vi "Main FPGA 5-axis with Limits and changes.vi"() -> ()   [LabVIEW 2013]
uses:
  <vilib>/Motion/MotorControl/_s/nism.interpretControlRegister.stateTransition.ctl
  <vilib>/Platform/TimedLoop/XDataNode/timing_clust.ctl
  <vilib>/Platform/TimedLoop/XDataNode/nitl_modes.ctl
  <vilib>/Platform/TimedLoop/XDataNode/wakeup.ctl
  <vilib>/Motion/MotorControl/_s/nism.digitalInputs.portA.ctl
  <vilib>/rvi/Emulation/niFpgaSctlEmulationGetInTimedLoop.vi
  <vilib>/rvi/Emulation/niFpgaEmulationReportErrorSimple.vi
  <vilib>/rvi/Emulation/niFpgaGetClockAttributes.vi
  <vilib>/rvi/Emulation/niFpgaCriticalErrorInLSC.vi
  Global FPGA.vi
  <vilib>/rvi/eio/common/nirviEmuTemplateMethod_errors.vi
  <vilib>/Motion/SoftMotion/Synchronization/nism.rioScan.generateSyncScan.vi
  <vilib>/rvi/Emulation/niFpgaProcessEmulError.vi
  <vilib>/Motion/MotorControl/_s/nism.interpretControlRegister.indexed.vi
  <vilib>/Motion/MotorControl/_s/nism.generateStatusRegister.indexed.vi
  <vilib>/Motion/MotorControl/_s/nism.mdo.read.dio.portA.2.vi
  <vilib>/Motion/MotorControl/_s/nism.mdo.read.positionLoopSyncData.vi
  <vilib>/Motion/MotorControl/_s/nism.mdo.read.splineData.vi
  <vilib>/Motion/MotorControl/_s/nism.splineInterpolation.fxp.3.index.vi
  <vilib>/Motion/MotorControl/_s/nism.mdo.handler.indexed.vi
  <vilib>/Motion/MotorControl/_s/nism.digitalFilter.u8.vi
  <vilib>/Motion/MotorControl/_s/nism.interpretDIOControl.portA.single.2.vi
  <vilib>/Motion/MotorControl/_s/nism.generateDIOStatus.portA.single.vi
  <vilib>/Platform/TimedLoop/XDataNode/XDataNode.xnode
  <vilib>/eio/EIONode/EIONode.xnode
  <vilib>/Motion/MotorControl/NI_SoftMotion_MotorControlIP.lvlib
  <vilib>/Platform/TimedLoop/XDataNode/XDNodeRunTimeDep.lvlib
  <vilib>/Motion/SoftMotion/Synchronization/NI_SoftMotion_Synchronization.lvlib
panel:
  in  "Axis Digital Inputs (U8)":u8[](array[numeric])=[0, 0, 0, 0, 0, 0, 0, 0]
  out "Axis Positions":fxp<+/-,64,32>[](array[numeric])
  in  "STEP or CW? (T=STEP)":bool
  out "Drive Enable":bool[](array[boolean])
  in  "Enable Watchdog":bool
  in  "Pet Watchdog":bool
  in  "Watchdog Timeout Period (ticks)":u64=40000000 format="%.0p"
  out "Watchdog Timed Out?":bool
  out "Time Since Last Pet":u64
  in  "Enable value":bool
  in  "Drive Enable override?":bool
  out "State":T1=enum."Start --> Initializing" caption="state transition"
  in  "Sync Value":bool
  in  "Sync Enable override?":bool
  in  "Invert direction?":bool
  out "Sync is Fault":bool
  out "Sync is Locked":bool
  in  "minimum pulse":u16=40
  # "Synchronization Loop"
  # "Control Status Loop"
  # "Notes: \n1. This VI provides the communication interface between the NI SoftMotion Engine and the LabVIEW FPGA Module. You must compile this VI for a specific FPGA target before use. After compiling, run the VI before running any of the Express VI examples. For information on moving this example to another FPGA target, refer to ni.com/info and enter info code fpgaex.\n\n2. Only use the Reset Axis button if you are unable to communicate with the axis by any other means. This button resets the device state machine and other VIs to a known state. After resetting the axis, switch the NI Scan Engine from Active Mode to Configuration Mode, then back to Active Mode, before attempting to enable the axis."
  # "(These two buttons \nare for testing\npurposes.)"
  # "(These two buttons \nare for testing\npurposes.)"
  # "Step/Direction Loop"
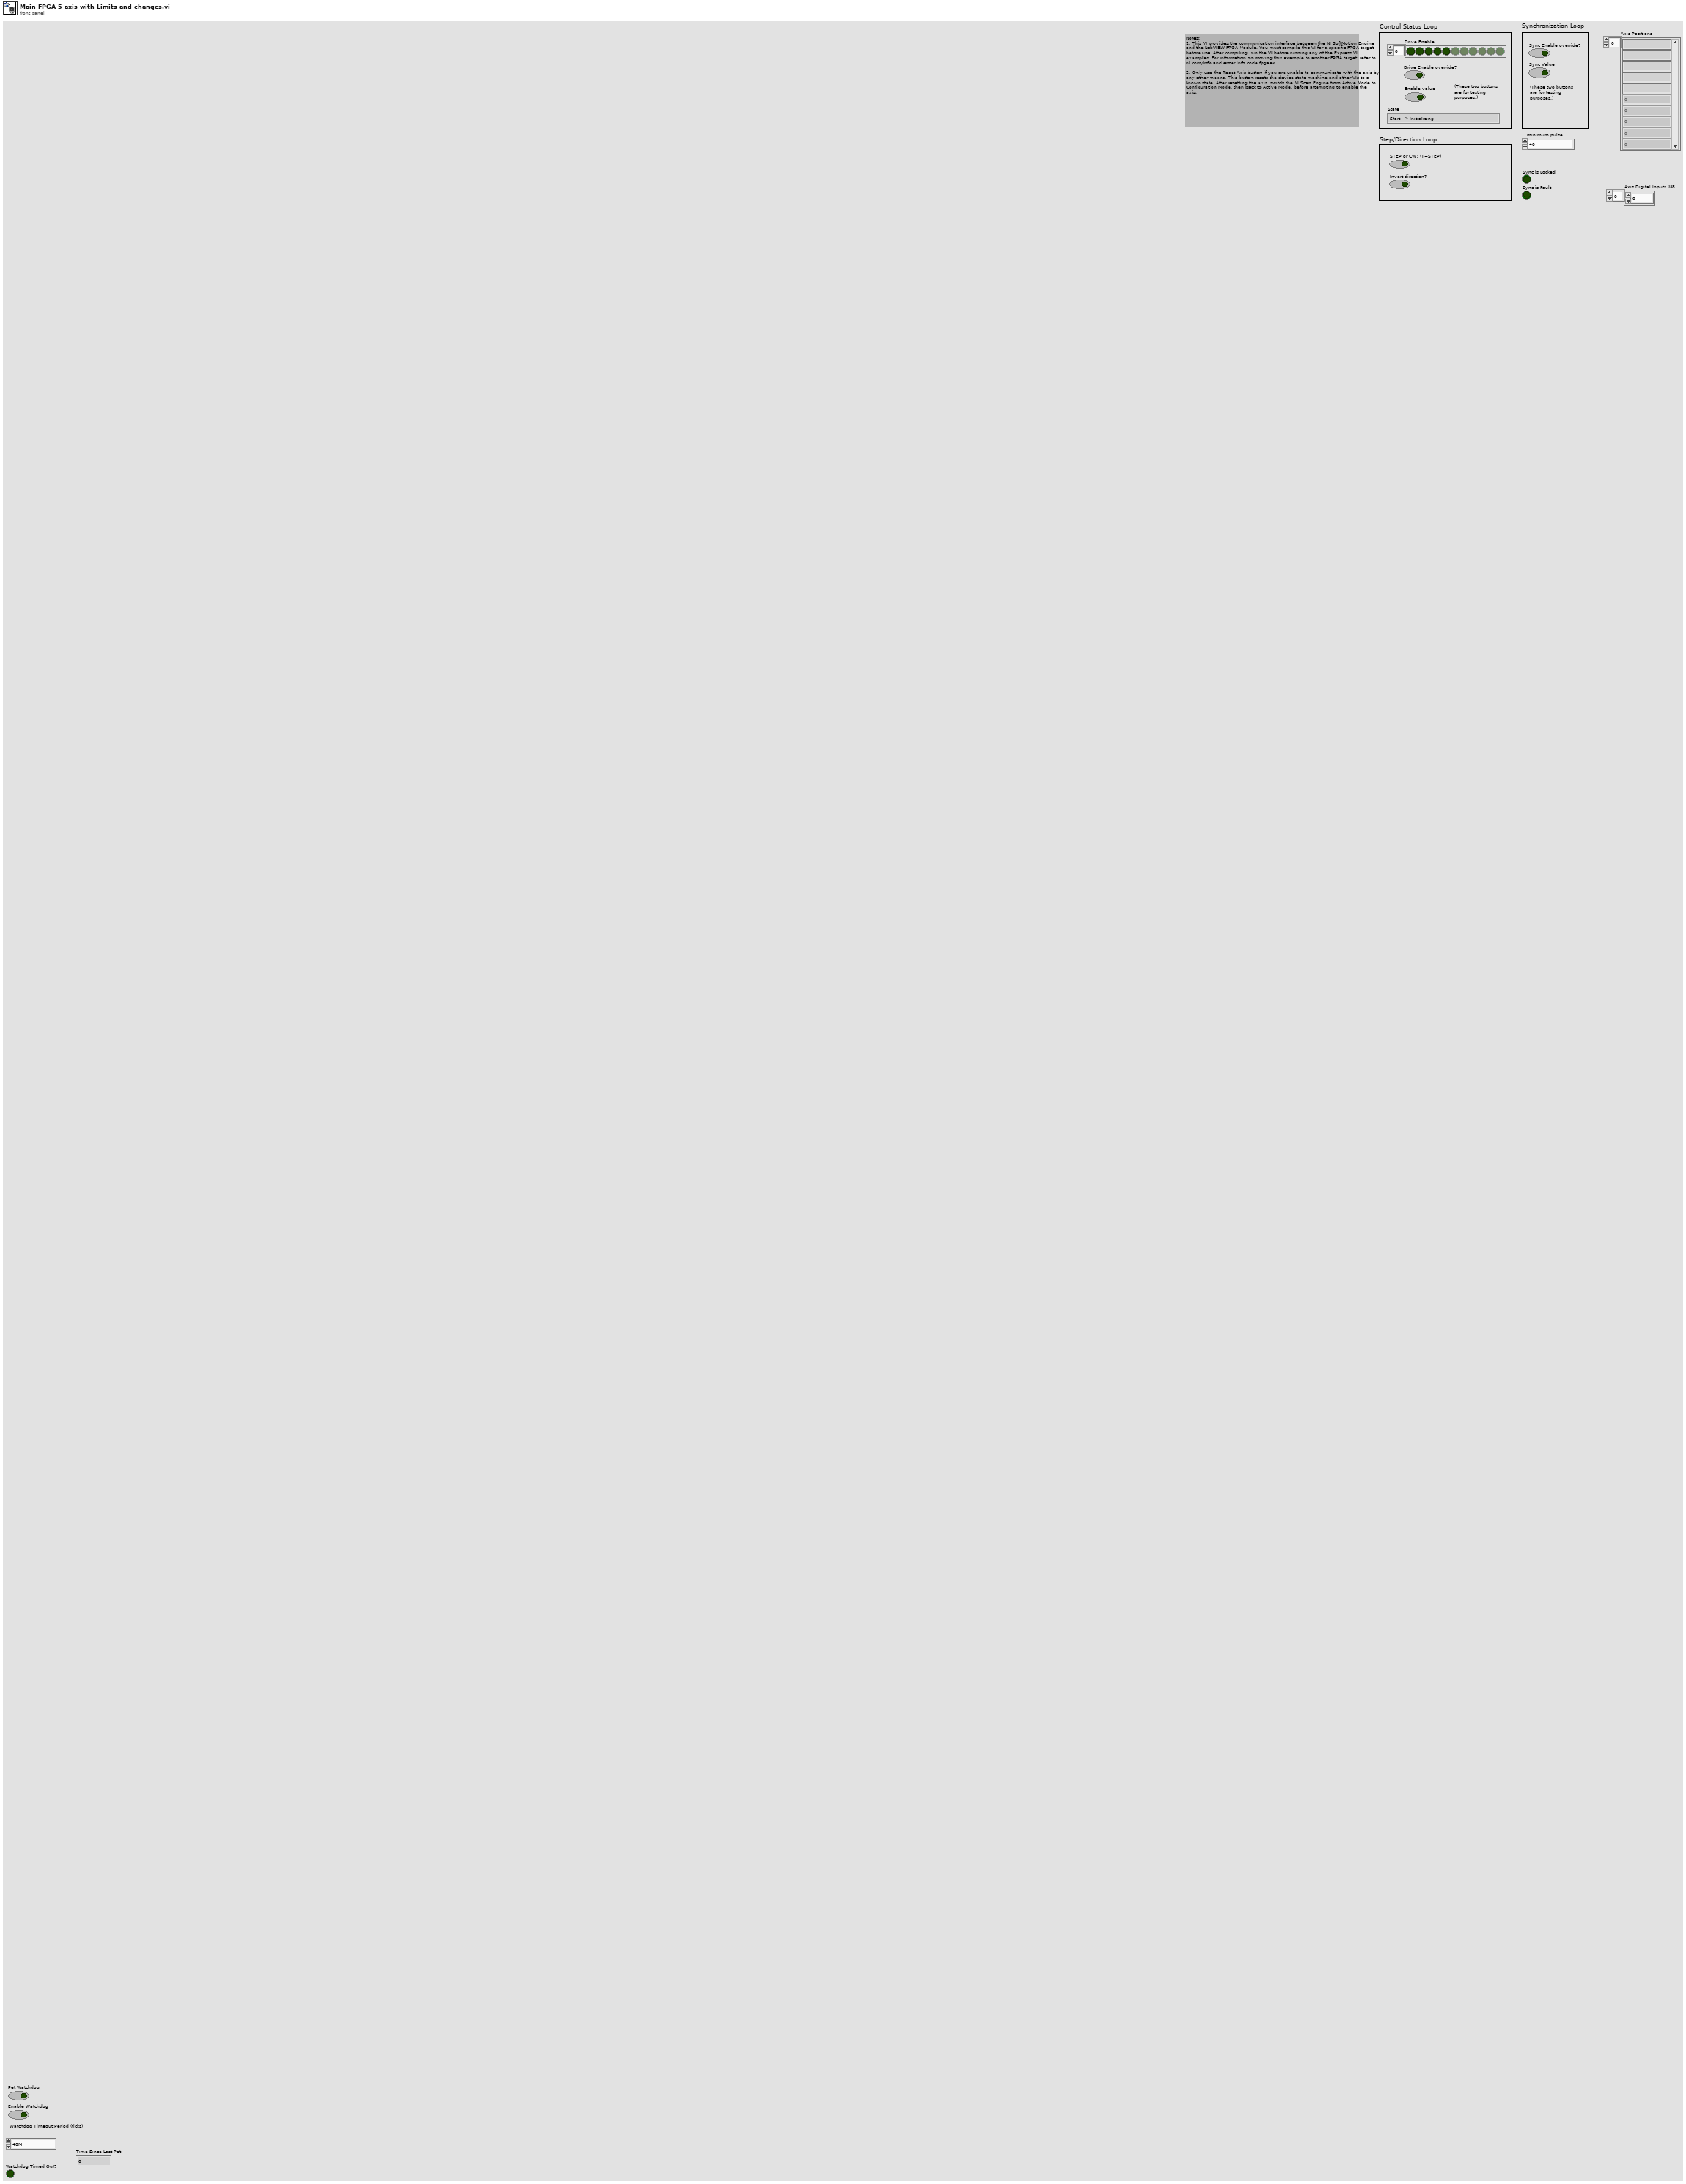
[diagram p1: front panel]
types:
  T1 = typedef "NI_SoftMotion_MotorControlIP.lvlib/nism.interpretControlRegister.stateTransition.ctl" = enum8{"Invalid", "Start --> Initializing", "Initializing --> Disabled", "Disabled --> Ready To Switch On", "Ready To Switch On --> Switched On", "Ready To Switch On --> Disable", "Switched On --> Operation Enable", "Switched On --> Ready To Switch On", "Switched On --> Disabled", "Operation Enable --> Switched On", "Operation Enable --> Ready To Switch On", "Operation Enable --> Disabled", "Fault --> Disabled", "Any --> Fault", "None"}
  T2 = typedef "NI_SoftMotion_MotorControlIP.lvlib/nism.dio.portA.config.2.ctl" = cluster{"digital filter (us)":u16[], "safe state":enum16{"Low", "High", "No Change"}[]}
  T3 = typedef "NI_SoftMotion_MotorControlIP.lvlib/nism.mdo.splineData.ctl" = cluster{"spline type":T4, "traj per/spline per":u16, "spline per/traj per":fxp<+,32,0>}
  T4 = typedef "nism.splineInterpolation.type.ctl" = u16
  T5 = typedef "NI_SoftMotion_Synchronization.lvlib/nism.softmotionScan.timerConfig.ctl" = cluster{"Target Period (clocks)":u16, "Host Period / Target Period":u16}
  T6 = typedef "NI_SoftMotion_Synchronization.lvlib/nism.softmotionScan.timerControl.ctl" = cluster{"SM Scan":bool, "SM Scan Count":u32, "SM Scan Enabled":bool}
  T7 = typedef "XDNodeRunTimeDep.lvlib/timing_clust.ctl" = cluster{"Expected End [f-1]":u64, "Actual End [f-1]":u64, "Finished Late? [f-1]":bool, "Expected End [i-1]":u64, "Actual End [i-1]":u64, "Finished Late? [i-1]":bool, "Expected Start [i]":u64, "Actual Start [i]":u64, "Expected Start [f]":u64, "Actual Start [f]":u64, "Source Name":string, "Structure Name":string, "Period":i64, "Deadline":i64, "Offset":i64, "Start":i64, "Priority":i32, "Timeout":i32, "Mode":T8, "Wakeup Reason":T9, "Error":errorcluster, "Source Type":string, "Secondary Source Type":string, "Global End Time":u64, "Global Start Time":u64, "Frame Duration":u64, "Iteration Duration":u64, "Assigned CPU":i32, "I/O Scan Engine Mode":u32}
  T8 = typedef "XDNodeRunTimeDep.lvlib/nitl_modes.ctl" = enum32{"No Change", "Process missed periods, maintain original phase", "Discard missed periods, maintain original phase", "Process missed periods, ignore original phase", "Discard missed periods, ignore original phase"}
  T9 = typedef "XDNodeRunTimeDep.lvlib/wakeup.ctl" = enum32{"Normal", "Aborted", "Asynchronous wakeup", "Timing source error", "Timed loop error", "Timeout"}
  T10 = typedef "NI_SoftMotion_MotorControlIP.lvlib/nism.digitalInputs.portA.ctl" = cluster{"reverse limit":bool, "forward limit":bool, "home switch":bool, "digital input 0":bool, "digital input 1":bool, "digital input 2":bool, "digital input 3":bool}
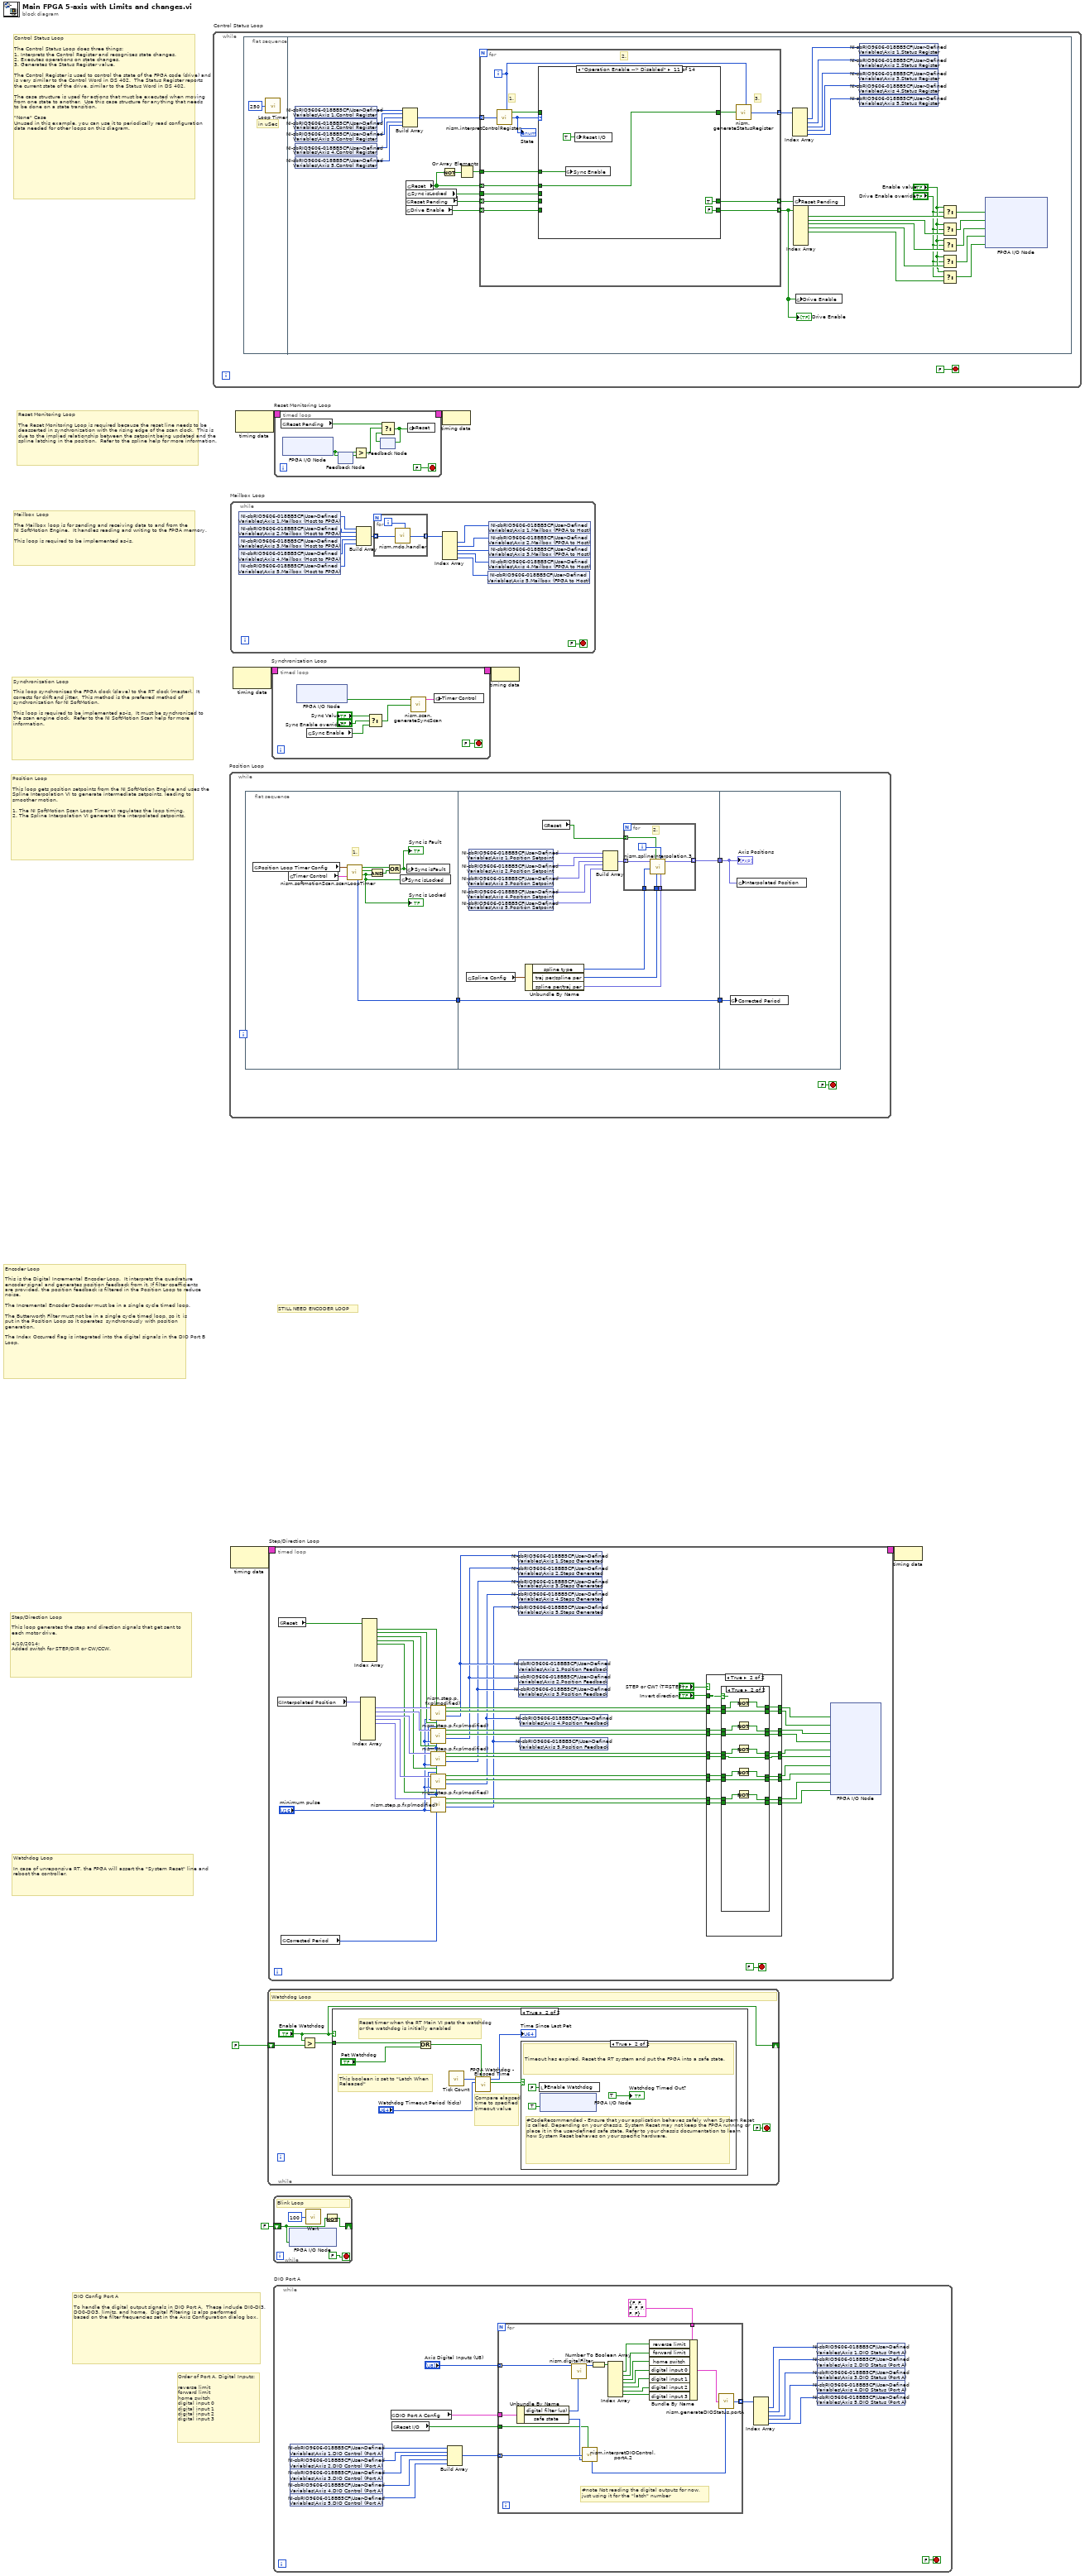
[diagram p0: block diagram]
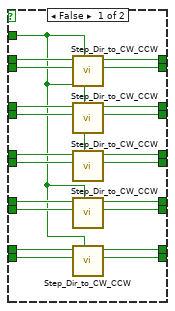
[diagram p4: hidden frame]
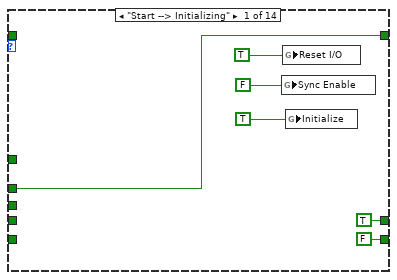
[diagram p6: hidden frame]
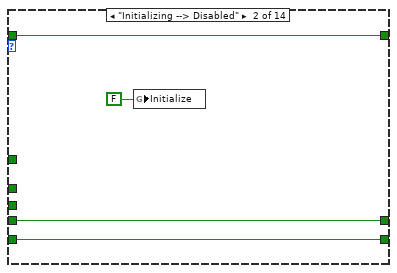
[diagram p7: hidden frame]
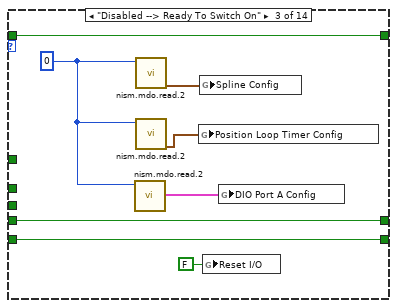
[diagram p8: hidden frame]
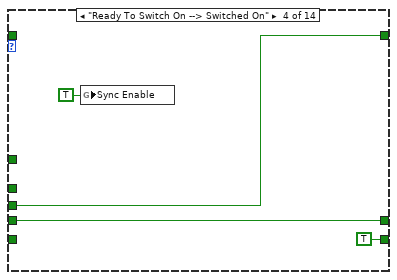
[diagram p9: hidden frame]
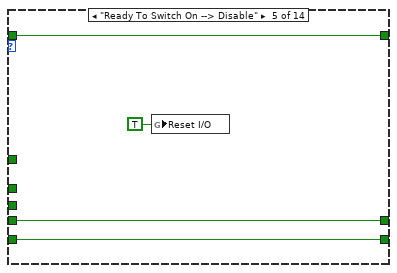
[diagram p10: hidden frame]
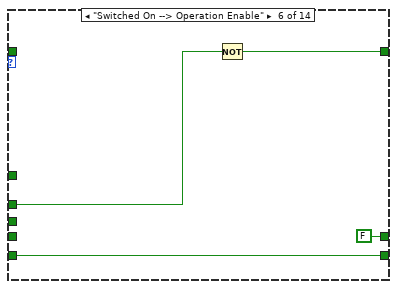
[diagram p11: hidden frame]
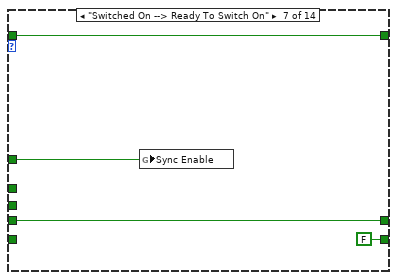
[diagram p12: hidden frame]
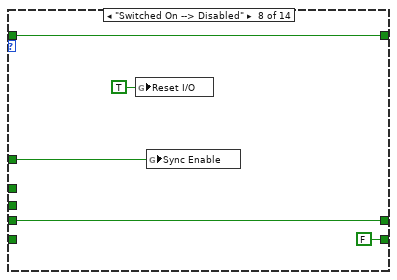
[diagram p13: hidden frame]
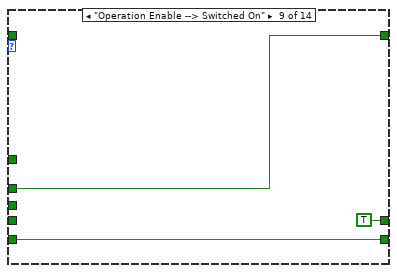
[diagram p14: hidden frame]
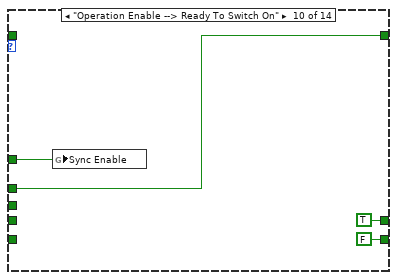
[diagram p15: hidden frame]
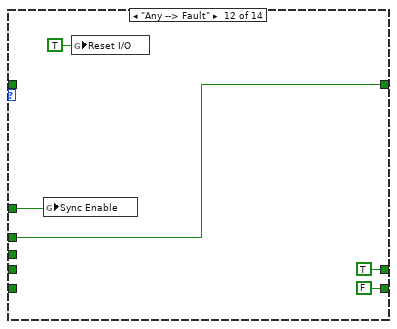
[diagram p16: hidden frame]
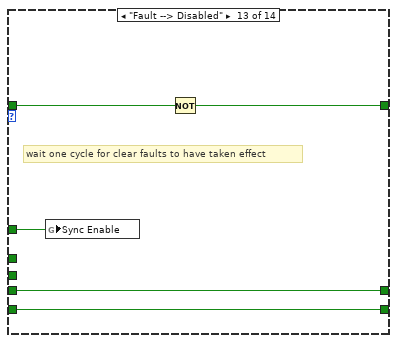
[diagram p17: hidden frame]
diagram:
  # "STILL NEED ENCODER LOOP"
  # "DIO Config Port A\n\nTo handle the digital output signals in DIO Port A.  These include DI0-DI3, DO0-DO3, limits, and home.  Digital Filtering is also performed\nbased on the filter frequencies set in the Axis Configuration dialog box."
  # "Order of Port A, Digital Inputs:\n\nreverse limit\nforward limit\nhome switch\ndigital input 0\ndigital input 1\ndigital input 2\ndigital input 3"
  # "Encoder Loop\n\nThis is the Digital Incremental Encoder Loop.  It interprets the quadrature encoder signal and generates position feedback from it. If filter coefficients are provided, the position feedback is filtered in the Position Loop to reduce noise.\n\nThe Incremental Encoder Decoder must be in a single cycle timed loop.\n\nThe Butterworth Filter must not be in a single cycle timed loop, so it  is\nput in the Position Loop so it operates  synchronously with position generation.\n\nThe Index Occurred flag is integrated into the digital signals in the DIO Port B Loop."
  # "Watchdog Loop\n\nIn case of unreponsive RT, the FPGA will assert the \"System Reset\" line and reboot the controller."
  # "Step/Direction Loop\n\nThis loop generates the step and direction signals that get sent to \neach motor drive.\n\n4/10/2014:\nAdded switch for STEP/DIR or CW/CCW."
  # "Position Loop\n\nThis loop gets position setpoints from the NI SoftMotion Engine and uses the Spline Interpolation VI to generate intermediate setpoints, leading to smoother motion.\n\n1. The NI SoftMotion Scan Loop Timer VI regulates the loop timing. \n2. The Spline Interpolation VI generates the interpolated setpoints."
  # "Synchronization Loop\n\nThis loop synchronizes the FPGA clock (slave) to the RT clock (master).  It corrects for drift and jitter.  This method is the preferred method of synchronization for NI SoftMotion.\n\nThis loop is required to be implemented as-is.  It must be synchronized to the scan engine clock.  Refer to the NI SoftMotion Scan help for more information."
  # "Mailbox Loop\n\nThe Mailbox loop is for sending and receiving data to and from the \nNI SoftMotion Engine.  It handles reading and writing to the FPGA memory.\n\nThis loop is required to be implemented as-is."
  # "Reset Monitoring Loop\n\nThe Reset Monitoring Loop is required because the reset line needs to be deasserted in synchronization with the rising edge of the scan clock.  This is due to the implied relationship between the setpoint being updated and the spline latching in the position.  Refer to the spline help for more information."
  # "Control Status Loop\n\nThe Control Status Loop does three things:\n1. Interprets the Control Register and recognizes state changes.\n2. Executes operations on state changes.\n3. Generates the Status Register value.\n\nThe Control Register is used to control the state of the FPGA code (drive) and is very similar to the Control Word in DS 402.  The Status Register reports the current state of the drive, similar to the Status Word in DS 402.\n\nThe case structure is used for actions that must be executed when moving from one state to another.  Use this case structure for anything that needs to be done on a state transition.\n\n\"None\" Case\nUnused in this example, you can use it to periodically read configuration data needed for other loops on this diagram."
  n1 = while "Control Status Loop" {
    stop <- FALSE stop-if-true
    n2 = flat-sequence {
      frame #0 {
        # "in uSec"
        n3 = call "Loop Timer"("Count(uSec)"=u32 250) -> ()  [unwired: 1 out]
      }
      frame #1 {
        n4 = shared-variable "NI-sbRIO9606-018BB5CF\\User-Defined Variables\\Axis 1.Control Register"() -> (w32:u32)  [unwired: 1 in, 1 out]
        n5 = shared-variable "NI-sbRIO9606-018BB5CF\\User-Defined Variables\\Axis 2.Control Register"() -> (w31:u32)  [unwired: 1 in, 1 out]
        n6 = shared-variable "NI-sbRIO9606-018BB5CF\\User-Defined Variables\\Axis 3.Control Register"() -> (w30:u32)  [unwired: 1 in, 1 out]
        n7 = shared-variable "NI-sbRIO9606-018BB5CF\\User-Defined Variables\\Axis 4.Control Register"() -> (w29:u32)  [unwired: 1 in, 1 out]
        n8 = shared-variable "NI-sbRIO9606-018BB5CF\\User-Defined Variables\\Axis 5.Control Register"() -> (w28:u32)  [unwired: 1 in, 1 out]
        n9 = Build Array(w32, w31, w30, w29, w28) -> (w41:u32[])
        n10 = global read "Global FPGA.vi" "Reset Pending"() -> (w36:bool[])
        n11 = global read "Global FPGA.vi" "Drive Enable"() -> (w35:bool[])
        n12 = global read "Global FPGA.vi" "Reset"() -> (w37:bool[])
        n13 = global read "Global FPGA.vi" "Sync isLocked"() -> (w42:bool)
        n14 = Not(x=w37) -> (.not. x?=w39:bool[])
        n15 = Or Array Elements(Boolean array=w39) -> (logical OR=w38:bool)
        n16 = for {
          tunnel: w37 -> [w50] mode=indexing
          tunnel: w42 -> [w49]
          tunnel: w41 -> [w51] mode=indexing
          tunnel: [w48] -> w33 mode=indexing
          tunnel: [w47] -> w40 mode=indexing
          tunnel: [w46] -> w34 mode=indexing
          tunnel: w38 -> [w45]
          tunnel: w36 -> [w44] mode=indexing
          tunnel: w35 -> [w43] mode=indexing
          i -> [w52]
          # "3."
          # "2."
          # "1."
          n17 = call-poly <vilib>:"nism.interpretControlRegister.vi"("control register"=w51, "axis index"=w52) -> ("transition occurred"=w53:bool, "state transition"=w54:T1)  [unwired: 6 in]
          "State" <- w54
          n18 = case shown="\"Operation Enable --> Disabled\"" w54 {
            tunnel: w53 -> [_ w65 w73 _ w81 _ w89 w94 _ _ _ _ w116 _]
            tunnel: [w61 w65 w73 w75 w81 w85 w89 w94 w96 w99 w104 w109 w115 _] -> w55
            tunnel: w50 -> [w61 _ _ _ _ w84 _ _ w96 w99 w104 w109 _ _]
            tunnel: w49 -> [_ _ _ w75 _ _ _ _ _ _ _ _ _ _]
            tunnel: [TRUE ("Write.Reset Pending") w64 w70 w74 w80 FALSE ("Write.Reset Pending") w86 w91 TRUE ("Write.Reset Pending") TRUE ("Write.Reset Pending") TRUE ("Write.Reset Pending") TRUE ("Write.Reset Pending") w113 w118] -> w47
            tunnel: [FALSE ("Write.Drive Enable") w63 w69 TRUE ("Write.Drive Enable") w79 w82 FALSE ("Write.Drive Enable") FALSE ("Write.Drive Enable") w95 FALSE ("Write.Drive Enable") FALSE ("Write.Drive Enable") FALSE ("Write.Drive Enable") w112 w117] -> w46
            tunnel: w45 -> [_ _ _ _ _ _ w87 w92 _ w98 w103 w108 w114 _]
            tunnel: w44 -> [_ w64 w70 w74 w80 _ w86 w91 _ _ _ _ w113 w118]
            tunnel: w43 -> [_ w63 w69 _ w79 w82 _ _ w95 _ _ _ w112 w117]
            frame "Start --> Initializing" {
              n19 = global write "Global FPGA.vi" "Sync Enable"(FALSE ("Sync Enable")) -> ()
              n20 = global write "Global FPGA.vi" "Reset I/O"(TRUE ("Reset I/O")) -> ()
              n21 = global write "Global FPGA.vi" "Initialize"(TRUE ("Reset I/O")) -> ()
            }
            frame "Initializing --> Disabled" {
              n22 = global write "Global FPGA.vi" "Initialize"(FALSE ("Reset I/O")) -> ()
            }
            frame "Disabled --> Ready To Switch On" {
              w67 = 0 ("axis index")
              n23 = call-poly <vilib>:"nism.mdo.read.2.vi"("axis index"=w67) -> ("dio config (port a)"=w66:T2)  [unwired: 10 in]
              n24 = call-poly <vilib>:"nism.mdo.read.2.vi"("axis index"=w67) -> ("spline"=w72:T3)  [unwired: 10 in]
              n25 = call-poly <vilib>:"nism.mdo.read.2.vi"("axis index"=w67) -> ("position loop sync"=w71:T5)  [unwired: 10 in]
              n26 = global write "Global FPGA.vi" "Position Loop Timer Config"(w71) -> ()
              n27 = global write "Global FPGA.vi" "Spline Config"(w72) -> ()
              n28 = global write "Global FPGA.vi" "Reset I/O"(FALSE ("Reset I/O")) -> ()
              n29 = global write "Global FPGA.vi" "DIO Port A Config"(w66) -> ()
            }
            frame "Ready To Switch On --> Switched On" {
              n30 = global write "Global FPGA.vi" "Sync Enable"(TRUE ("Sync Enable")) -> ()
            }
            frame "Ready To Switch On --> Disable" {
              n31 = global write "Global FPGA.vi" "Reset I/O"(TRUE ("Reset I/O")) -> ()
            }
            frame "Switched On --> Operation Enable" {
              n32 = Not(x=w84) -> (.not. x?=w85:bool)
            }
            frame "Switched On --> Ready To Switch On" {
              n33 = global write "Global FPGA.vi" "Sync Enable"(w87) -> ()
            }
            frame "Switched On --> Disabled" {
              n34 = global write "Global FPGA.vi" "Reset I/O"(TRUE ("Reset I/O")) -> ()
              n35 = global write "Global FPGA.vi" "Sync Enable"(w92) -> ()
            }
            frame "Operation Enable --> Switched On" {
            }
            frame "Operation Enable --> Ready To Switch On" {
              n36 = global write "Global FPGA.vi" "Sync Enable"(w98) -> ()
            }
            frame "Operation Enable --> Disabled" {
              n37 = global write "Global FPGA.vi" "Sync Enable"(w103) -> ()
              n38 = global write "Global FPGA.vi" "Reset I/O"(TRUE ("Reset I/O")) -> ()
            }
            frame "Any --> Fault" {
              n39 = global write "Global FPGA.vi" "Sync Enable"(w108) -> ()
              n40 = global write "Global FPGA.vi" "Reset I/O"(TRUE ("Reset I/O")) -> ()
            }
            frame "Fault --> Disabled" {
              # "wait one cycle for clear faults to have taken effect"
              n41 = global write "Global FPGA.vi" "Sync Enable"(w114) -> ()
              n42 = Not(x=w116) -> (.not. x?=w115:bool)
            }
            frame "None", Default {
            }
          }
          n43 = call-poly <vilib>:"nism.generateStatusRegister.vi"("transition success"=w55, "axis index"=w52) -> ("status register"=w48:u32)  [unwired: 7 in]
        }
        "Drive Enable" <- w34
        n44 = Index Array(array=w33) -> (element #1=w27:u32, element #2=w26:u32, element #3=w25:u32, element #4=w24:u32, element #5=w23:u32)  [unwired: 5 in]
        n45 = global write "Global FPGA.vi" "Reset Pending"(w40) -> ()
        n46 = Index Array(array=w34) -> (element #1=w22:bool, element #2=w20:bool, element #3=w18:bool, element #4=w16:bool, element #5=w14:bool)  [unwired: 8 in, 3 out]
        n47 = global write "Global FPGA.vi" "Drive Enable"(w34) -> ()
        n48 = shared-variable "NI-sbRIO9606-018BB5CF\\User-Defined Variables\\Axis 1.Status Register"(w27) -> ()  [unwired: 1 in, 1 out]
        n49 = shared-variable "NI-sbRIO9606-018BB5CF\\User-Defined Variables\\Axis 2.Status Register"(w26) -> ()  [unwired: 1 in, 1 out]
        n50 = shared-variable "NI-sbRIO9606-018BB5CF\\User-Defined Variables\\Axis 3.Status Register"(w25) -> ()  [unwired: 1 in, 1 out]
        n51 = shared-variable "NI-sbRIO9606-018BB5CF\\User-Defined Variables\\Axis 4.Status Register"(w24) -> ()  [unwired: 1 in, 1 out]
        n52 = shared-variable "NI-sbRIO9606-018BB5CF\\User-Defined Variables\\Axis 5.Status Register"(w23) -> ()  [unwired: 1 in, 1 out]
        n53 = Select(t="Enable value", s="Drive Enable override?", f=w22) -> (s? t:f=w21:bool)
        n54 = Select(t="Enable value", s="Drive Enable override?", f=w20) -> (s? t:f=w19:bool)
        n55 = Select(t="Enable value", s="Drive Enable override?", f=w18) -> (s? t:f=w17:bool)
        n56 = Select(t="Enable value", s="Drive Enable override?", f=w16) -> (s? t:f=w15:bool)
        n57 = Select(t="Enable value", s="Drive Enable override?", f=w14) -> (s? t:f=w13:bool)
        n58 = xnode "FPGA I/O Node"("Axis1_Servo On"=w21, "Axis2_Servo On"=w19, "Axis3_Servo On"=w17, "Axis4_Servo On"=w15, "Axis5_Servo On"=w13) -> ()  [unwired: 5 in, 5 out]
      }
    }
  }
  n59 = while "Position Loop" {
    stop <- FALSE stop-if-true
    n60 = flat-sequence {
      tunnel: [w123] -> w119
      tunnel: [w137] -> w121
      tunnel: [w136] -> w120
      tunnel: w119 -> [w136]
      tunnel: w121 -> [w151]
      tunnel: w120 -> [w152]
      frame #0 {
        # "1."
        n61 = global read "Global FPGA.vi" "Position Loop Timer Config"() -> (w125:T5)
        n62 = global read "Global FPGA.vi" "Timer Control"() -> (w124:T6)
        n63 = call <vilib>:"nism.softmotionScan.scanLoopTimer.vi"("Timer Control"=w124, "Timer Config"=w125) -> ("Scan Running?"=w127:bool, "Finished Late?"=w129:bool, "Fault Occurred?"=w130:bool, "Corrected Period"=w123:u16)  [unwired: 5 in, 1 out]
        "Sync is Locked" <- w127
        n64 = Compound Arithmetic op=AND(w129, w127) -> (w128:bool)
        n65 = Compound Arithmetic op=OR(w130, w128) -> (w126:bool)
        "Sync is Fault" <- w126
        n66 = global write "Global FPGA.vi" "Sync isLocked"(w127) -> ()
        n67 = global write "Global FPGA.vi" "Sync isFault"(w126) -> ()
      }
      frame #1 {
        n68 = global read "Global FPGA.vi" "Spline Config"() -> (w139:T3)
        n69 = shared-variable "NI-sbRIO9606-018BB5CF\\User-Defined Variables\\Axis 1.Position Setpoint"() -> (w135:fxp<+/-,64,32>)  [unwired: 1 in, 1 out]
        n70 = shared-variable "NI-sbRIO9606-018BB5CF\\User-Defined Variables\\Axis 2.Position Setpoint"() -> (w134:fxp<+/-,64,32>)  [unwired: 1 in, 1 out]
        n71 = shared-variable "NI-sbRIO9606-018BB5CF\\User-Defined Variables\\Axis 3.Position Setpoint"() -> (w133:fxp<+/-,64,32>)  [unwired: 1 in, 1 out]
        n72 = shared-variable "NI-sbRIO9606-018BB5CF\\User-Defined Variables\\Axis 4.Position Setpoint"() -> (w132:fxp<+/-,64,32>)  [unwired: 1 in, 1 out]
        n73 = shared-variable "NI-sbRIO9606-018BB5CF\\User-Defined Variables\\Axis 5.Position Setpoint"() -> (w131:fxp<+/-,64,32>)  [unwired: 1 in, 1 out]
        n74 = Unbundle By Name(w139) -> ("spline type"=w143:T4, "traj per/spline per"=w142:u16, "spline per/traj per"=w141:fxp<+,32,0>)
        n75 = global read "Global FPGA.vi" "Reset"() -> (w138:bool[])
        n76 = Build Array(w135, w134, w133, w132, w131) -> (w140:fxp<+/-,64,32>[])
        n77 = for {
          tunnel: w143 -> [w150]
          tunnel: w142 -> [w149]
          tunnel: w141 -> [w148]
          tunnel: w138 -> [w145] mode=indexing
          tunnel: w140 -> [w147] mode=indexing
          tunnel: [w144] -> w137 mode=indexing
          i -> [w146]
          # "2."
          n78 = call-poly <vilib>:"nism.splineInterpolation.3.vi"("1 / calls per sample"=w148, "index"=w146, "calls per sample"=w149, "reset"=w145, "spline type"=w150, "x"=w147) -> ("xi"=w144:fxp<+/-,64,32>)  [unwired: 5 in]
        }
      }
      frame #2 {
        n79 = global write "Global FPGA.vi" "Corrected Period"(w152) -> ()
        n80 = global write "Global FPGA.vi" "Interpolated Position"(w151) -> ()
        "Axis Positions" <- w151
      }
    }
  }
  n81 = while "Mailbox Loop" {
    stop <- FALSE stop-if-true
    n82 = shared-variable "NI-sbRIO9606-018BB5CF\\User-Defined Variables\\Axis 1.Mailbox (Host to FPGA)"() -> (w162:u64)  [unwired: 1 in, 1 out]
    n83 = shared-variable "NI-sbRIO9606-018BB5CF\\User-Defined Variables\\Axis 2.Mailbox (Host to FPGA)"() -> (w161:u64)  [unwired: 1 in, 1 out]
    n84 = shared-variable "NI-sbRIO9606-018BB5CF\\User-Defined Variables\\Axis 3.Mailbox (Host to FPGA)"() -> (w160:u64)  [unwired: 1 in, 1 out]
    n85 = shared-variable "NI-sbRIO9606-018BB5CF\\User-Defined Variables\\Axis 4.Mailbox (Host to FPGA)"() -> (w159:u64)  [unwired: 1 in, 1 out]
    n86 = shared-variable "NI-sbRIO9606-018BB5CF\\User-Defined Variables\\Axis 5.Mailbox (Host to FPGA)"() -> (w158:u64)  [unwired: 1 in, 1 out]
    n87 = Build Array(w162, w161, w160, w159, w158) -> (w164:u64[])
    n88 = for {
      tunnel: w164 -> [w168] mode=indexing
      tunnel: [w167] -> w163 mode=indexing
      i -> [w166]
      n89 = call-poly <vilib>:"nism.mdo.handler.vi"("mbox (host to fpga)"=w168, "axis index"=w166) -> ("mbox (fpga to host)"=w167:u64)  [unwired: 7 in]
    }
    n90 = Index Array(array=w163) -> (element #1=w157:u64, element #2=w156:u64, element #3=w155:u64, element #4=w154:u64, element #5=w153:u64)  [unwired: 5 in]
    n91 = shared-variable "NI-sbRIO9606-018BB5CF\\User-Defined Variables\\Axis 5.Mailbox (FPGA to Host)"(w153) -> ()  [unwired: 1 in, 1 out]
    n92 = shared-variable "NI-sbRIO9606-018BB5CF\\User-Defined Variables\\Axis 1.Mailbox (FPGA to Host)"(w157) -> ()  [unwired: 1 in, 1 out]
    n93 = shared-variable "NI-sbRIO9606-018BB5CF\\User-Defined Variables\\Axis 2.Mailbox (FPGA to Host)"(w156) -> ()  [unwired: 1 in, 1 out]
    n94 = shared-variable "NI-sbRIO9606-018BB5CF\\User-Defined Variables\\Axis 3.Mailbox (FPGA to Host)"(w155) -> ()  [unwired: 1 in, 1 out]
    n95 = shared-variable "NI-sbRIO9606-018BB5CF\\User-Defined Variables\\Axis 4.Mailbox (FPGA to Host)"(w154) -> ()  [unwired: 1 in, 1 out]
  }
  n96 = node-c288() -> (w8:T7)  [unwired: 1 in]
  n97 = node-c288() -> (w6:T7)  [unwired: 1 in]
  n98 = node-c288() -> (w4:T7)  [unwired: 1 in]
  n99 = while "RT Watchdog Loop" {
    shift-right: ["Enable Watchdog"] -> _
    shift-left: FALSE ("Enable RT Watchdog") -> [w172]
    stop <- FALSE stop-if-true
    # "Watchdog Loop"
    n100 = Greater?(x="Enable Watchdog", y=w172) -> (0:w169:bool)
    n101 = case shown="True" "Enable Watchdog" {
      tunnel: w169 -> [_ w175]
      frame False {
        # "This loop has to be explicitly enabled from the RT Main VI.  This reduces the possiblity of an endless reboot cycle."
      }
      frame True {
        # "This boolean is set to \"Latch When Released\""
        # "Compare elapsed time to specified timeout value"
        # "Reset timer when the RT Main VI pets the watchdog or the watchdog is initially enabled"
        n102 = Or(x=w175, y="Pet Watchdog") -> (x .or. y?=w174:bool)
        n103 = call "Tick Count"() -> ("Tick Count(Ticks)"=w178:u32)
        n104 = call "FPGA Watchdog - Elapsed Time.vi"("Reset"=w174, "Timeout Period"="Watchdog Timeout Period (ticks)", "Current Time"=w178) -> ("Timeout"=w173:bool, "Elapsed Time"=→"Time Since Last Pet":u64)  [unwired: 7 in]
        n105 = case shown="True" w173 {
          frame False {
            # "Timeout has not expired."
          }
          frame True {
            # "#CodeRecommended - Ensure that your application behaves safely when System Reset is called. Depending on your chassis, System Reset may not keep the FPGA running or place it in the user-defined safe state. Refer to your chassis documentation to learn how System Reset behaves on your specific hardware."
            # "Timeout has expired. Reset the RT system and put the FPGA into a safe state."
            n106 = local write "Enable Watchdog"(FALSE ("Enable RT Watchdog")) -> ()
            n107 = xnode "FPGA I/O Node"("System Reset"=TRUE ("RT Reset on Watchdog Failure?")) -> ()  [unwired: 1 in, 1 out]
            "Watchdog Timed Out?" <- TRUE ("Watchdog Timed Out?")
          }
        }
      }
    }
  }
  n108 = timed-loop "Step/Direction Loop" {
    timing: w8 -> [_]
    timing-out: [_] -> w7
    stop <- FALSE stop-if-true
    n109 = global read "Global FPGA.vi" "Interpolated Position"() -> (w223:fxp<+/-,64,32>[])
    n110 = global read "Global FPGA.vi" "Reset"() -> (w217:bool[])
    n111 = global read "Global FPGA.vi" "Corrected Period"() -> (w183:u16)
    n112 = Index Array(array=w223) -> (element #1=w222:fxp<+/-,64,32>, element #2=w221:fxp<+/-,64,32>, element #3=w220:fxp<+/-,64,32>, element #4=w219:fxp<+/-,64,32>, element #5=w218:fxp<+/-,64,32>)  [unwired: 9 in, 4 out]
    n113 = Index Array(array=w217) -> (element #1=w216:bool, element #2=w215:bool, element #3=w214:bool, element #4=w213:bool, element #5=w212:bool)  [unwired: 9 in, 4 out]
    n114 = call "nism.step.p.fxp(modified).vi"("calls per sample"=w183, "reset"=w216, "minimum pulse"="minimum pulse", "position setpoint"=w222) -> ("steps generated"=w188:i32, "step"=w210:bool, "direction"=w211:bool)  [unwired: 4 in, 1 out]
    n115 = call "nism.step.p.fxp(modified).vi"("calls per sample"=w183, "reset"=w215, "minimum pulse"="minimum pulse", "position setpoint"=w221) -> ("steps generated"=w187:i32, "step"=w208:bool, "direction"=w209:bool)  [unwired: 4 in, 1 out]
    n116 = call "nism.step.p.fxp(modified).vi"("calls per sample"=w183, "reset"=w214, "minimum pulse"="minimum pulse", "position setpoint"=w220) -> ("steps generated"=w186:i32, "step"=w206:bool, "direction"=w207:bool)  [unwired: 4 in, 1 out]
    n117 = call "nism.step.p.fxp(modified).vi"("calls per sample"=w183, "reset"=w213, "minimum pulse"="minimum pulse", "position setpoint"=w219) -> ("steps generated"=w185:i32, "step"=w204:bool, "direction"=w205:bool)  [unwired: 4 in, 1 out]
    n118 = call "nism.step.p.fxp(modified).vi"("calls per sample"=w183, "reset"=w212, "minimum pulse"="minimum pulse", "position setpoint"=w218) -> ("steps generated"=w184:i32, "step"=w202:bool, "direction"=w203:bool)  [unwired: 4 in, 1 out]
    n119 = shared-variable "NI-sbRIO9606-018BB5CF\\User-Defined Variables\\Axis 1.Steps Generated"(w188) -> ()  [unwired: 1 in, 1 out]
    n120 = shared-variable "NI-sbRIO9606-018BB5CF\\User-Defined Variables\\Axis 2.Steps Generated"(w187) -> ()  [unwired: 1 in, 1 out]
    n121 = shared-variable "NI-sbRIO9606-018BB5CF\\User-Defined Variables\\Axis 3.Steps Generated"(w186) -> ()  [unwired: 1 in, 1 out]
    n122 = shared-variable "NI-sbRIO9606-018BB5CF\\User-Defined Variables\\Axis 4.Steps Generated"(w185) -> ()  [unwired: 1 in, 1 out]
    n123 = shared-variable "NI-sbRIO9606-018BB5CF\\User-Defined Variables\\Axis 5.Steps Generated"(w184) -> ()  [unwired: 1 in, 1 out]
    n124 = shared-variable "NI-sbRIO9606-018BB5CF\\User-Defined Variables\\Axis 1.Position Feedback"(w188) -> ()  [unwired: 1 in, 1 out]
    n125 = shared-variable "NI-sbRIO9606-018BB5CF\\User-Defined Variables\\Axis 2.Position Feedback"(w187) -> ()  [unwired: 1 in, 1 out]
    n126 = shared-variable "NI-sbRIO9606-018BB5CF\\User-Defined Variables\\Axis 3.Position Feedback"(w186) -> ()  [unwired: 1 in, 1 out]
    n127 = shared-variable "NI-sbRIO9606-018BB5CF\\User-Defined Variables\\Axis 4.Position Feedback"(w185) -> ()  [unwired: 1 in, 1 out]
    n128 = shared-variable "NI-sbRIO9606-018BB5CF\\User-Defined Variables\\Axis 5.Position Feedback"(w184) -> ()  [unwired: 1 in, 1 out]
    n129 = case shown="True" "STEP or CW? (T=STEP)" {
      tunnel: w211 -> [w245 w265]
      tunnel: w210 -> [w244 w255]
      tunnel: w209 -> [w243 w263]
      tunnel: w208 -> [w242 w253]
      tunnel: w207 -> [w241 w261]
      tunnel: w206 -> [w240 w251]
      tunnel: w205 -> [w239 w259]
      tunnel: w204 -> [w238 w249]
      tunnel: w203 -> [w237 w257]
      tunnel: w202 -> [w236 w247]
      tunnel: "Invert direction?" -> [w225 w266]
      tunnel: [w235 w264] -> w200
      tunnel: [w234 w254] -> w191
      tunnel: [w233 w262] -> w199
      tunnel: [w232 w252] -> w198
      tunnel: [w231 w260] -> w197
      tunnel: [w230 w250] -> w196
      tunnel: [w229 w258] -> w195
      tunnel: [w228 w248] -> w194
      tunnel: [w227 w256] -> w193
      tunnel: [w226 w246] -> w192
      frame False {
        n130 = call "Step_Dir_to_CW_CCW.vi"("invert"=w225, "step"=w244, "direction"=w245) -> ("CCW"=w234:bool, "CW"=w235:bool)  [unwired: 7 in]
        n131 = call "Step_Dir_to_CW_CCW.vi"("invert"=w225, "step"=w242, "direction"=w243) -> ("CCW"=w232:bool, "CW"=w233:bool)  [unwired: 7 in]
        n132 = call "Step_Dir_to_CW_CCW.vi"("invert"=w225, "step"=w240, "direction"=w241) -> ("CCW"=w230:bool, "CW"=w231:bool)  [unwired: 7 in]
        n133 = call "Step_Dir_to_CW_CCW.vi"("invert"=w225, "step"=w238, "direction"=w239) -> ("CCW"=w228:bool, "CW"=w229:bool)  [unwired: 7 in]
        n134 = call "Step_Dir_to_CW_CCW.vi"("invert"=w225, "step"=w236, "direction"=w237) -> ("CCW"=w226:bool, "CW"=w227:bool)  [unwired: 7 in]
      }
      frame True {
        n135 = case shown="True" w266 {
          tunnel: w265 -> [w276 w291]
          tunnel: [w276 w290] -> w264
          tunnel: w263 -> [w274 w289]
          tunnel: [w274 w288] -> w262
          tunnel: w261 -> [w272 w287]
          tunnel: [w272 w286] -> w260
          tunnel: w259 -> [w270 w285]
          tunnel: [w270 w284] -> w258
          tunnel: w257 -> [w268 w283]
          tunnel: [w268 w282] -> w256
          tunnel: w255 -> [w275 w281]
          tunnel: [w275 w281] -> w254
          tunnel: w253 -> [w273 w280]
          tunnel: [w273 w280] -> w252
          tunnel: w251 -> [w271 w279]
          tunnel: [w271 w279] -> w250
          tunnel: w249 -> [w269 w278]
          tunnel: [w269 w278] -> w248
          tunnel: w247 -> [w267 w277]
          tunnel: [w267 w277] -> w246
          frame False {
          }
          frame True {
            n136 = Not(x=w291) -> (.not. x?=w290:bool)
            n137 = Not(x=w289) -> (.not. x?=w288:bool)
            n138 = Not(x=w287) -> (.not. x?=w286:bool)
            n139 = Not(x=w285) -> (.not. x?=w284:bool)
            n140 = Not(x=w283) -> (.not. x?=w282:bool)
          }
        }
      }
    }
    n141 = xnode "FPGA I/O Node"("Axis1_CW"=w200, "Axis1_CCW"=w191, "Axis2_CW"=w199, "Axis2_CCW"=w198, "Axis3_CW"=w197, "Axis3_CCW"=w196, "Axis4_CW"=w195, "Axis4_CCW"=w194, "Axis5_CW"=w193, "Axis5_CCW"=w192) -> ()  [unwired: 10 in, 10 out]
  }
  n142 = timed-loop "Synchronization Loop" {
    timing: w6 -> [_]
    timing-out: [_] -> w5
    stop <- FALSE stop-if-true
    n143 = xnode "FPGA I/O Node"() -> ("Scan Clock"=w298:bool)  [unwired: 1 in, 1 out]
    n144 = global read "Global FPGA.vi" "Sync Enable"() -> (w297:bool)
    n145 = Select(t="Sync Value", s="Sync Enable override?", f=w297) -> (s? t:f=w294:bool)
    n146 = call-poly <vilib>:"nism.scan.generateSyncScan.vi"("Scan Enable?"=w294, "Scan Clock"=w298) -> ("Timer Control"=w299:T6)  [unwired: 3 in]
    n147 = global write "Global FPGA.vi" "Timer Control"(w299) -> ()
  }
  n148 = while {
    shift-right: [w305] -> _
    shift-left: FALSE ("RT Reset on Watchdog Failure?") -> [w304]
    stop <- FALSE stop-if-true
    # "Blink Loop"
    n149 = xnode "FPGA I/O Node"("FPGA LED"=w304) -> ()  [unwired: 1 in, 1 out]
    n150 = call "Wait"("Count(mSec)"=u8 100) -> ()  [unwired: 1 out]
    n151 = Not(x=w304) -> (.not. x?=w305:bool)
  }
  n152 = while "DIO Port A" {
    stop <- FALSE stop-if-true
    n153 = shared-variable "NI-sbRIO9606-018BB5CF\\User-Defined Variables\\Axis 1.DIO Control (Port A)"() -> (w322:u32)  [unwired: 1 in, 1 out]
    n154 = shared-variable "NI-sbRIO9606-018BB5CF\\User-Defined Variables\\Axis 2.DIO Control (Port A)"() -> (w321:u32)  [unwired: 1 in, 1 out]
    n155 = shared-variable "NI-sbRIO9606-018BB5CF\\User-Defined Variables\\Axis 3.DIO Control (Port A)"() -> (w320:u32)  [unwired: 1 in, 1 out]
    n156 = shared-variable "NI-sbRIO9606-018BB5CF\\User-Defined Variables\\Axis 4.DIO Control (Port A)"() -> (w319:u32)  [unwired: 1 in, 1 out]
    n157 = shared-variable "NI-sbRIO9606-018BB5CF\\User-Defined Variables\\Axis 5.DIO Control (Port A)"() -> (w318:u32)  [unwired: 1 in, 1 out]
    n158 = global read "Global FPGA.vi" "DIO Port A Config"() -> (w308:T2)
    n159 = global read "Global FPGA.vi" "Reset I/O"() -> (w307:bool)
    n160 = Build Array(w322, w321, w320, w319, w318) -> (w317:u32[])
    n161 = for {
      tunnel: [w341] -> w316 mode=indexing
      tunnel: w317 -> [w340] mode=indexing
      tunnel: w308 -> [w330]
      tunnel: w307 -> [w328]
      tunnel: T10 {"reverse limit"=FALSE, "forward limit"=FALSE, "home switch"=FALSE, "digital input 0"=FALSE, "digital input 1"=FALSE, "digital input 2"=FALSE, "digital input 3"=FALSE} ("$(driveInterface.digitalInputs.shortName)") -> [w327]
      tunnel: "Axis Digital Inputs (U8)" -> [w324] mode=indexing
      # "#note Not reading the digital outputs for now,\njust using it for the \"latch\" number"
      n162 = Unbundle By Name(w330) -> ("digital filter (us)"=w338:u16[], "safe state"=w329:enum16{"Low", "High", "No Change"}[])
      n163 = call-poly <vilib>:"nism.digitalFilter.vi"("filter value (us)"=w338, "input signal"=w324) -> ("output signal"=w326:u8)  [unwired: 9 in]
      n164 = call-poly <vilib>:"nism.interpretDIOControl.portA.2.vi"("reset"=w328, "dio control(port a)"=w340, "safe state"=w329) -> ("reset latches"=w342:u8)  [unwired: 5 in, 1 out]
      n165 = Number To Boolean Array(number=w326) -> (Boolean array=w325:bool[])
      n166 = Index Array(array=w325) -> (element #1=w337:bool, element #2=w336:bool, element #3=w335:bool, element #4=w334:bool, element #5=w333:bool, element #6=w332:bool, element #7=w331:bool)  [unwired: 7 in]
      n167 = Bundle By Name(cluster=w327, "reverse limit"=w337, "forward limit"=w336, "home switch"=w335, "digital input 0"=w334, "digital input 1"=w333, "digital input 2"=w332, "digital input 3"=w331) -> (w339:T10)
      n168 = call-poly <vilib>:"nism.generateDIOStatus.portA.vi"("digital inputs"=w339, "reset latches"=w342) -> ("dio status(port a)"=w341:u32)  [unwired: 7 in]
    }
    n169 = Index Array(array=w316) -> (element #1=w315:u32, element #2=w314:u32, element #3=w313:u32, element #4=w312:u32, element #5=w311:u32)  [unwired: 5 in]
    n170 = shared-variable "NI-sbRIO9606-018BB5CF\\User-Defined Variables\\Axis 1.DIO Status (Port A)"(w315) -> ()  [unwired: 1 in, 1 out]
    n171 = shared-variable "NI-sbRIO9606-018BB5CF\\User-Defined Variables\\Axis 2.DIO Status (Port A)"(w314) -> ()  [unwired: 1 in, 1 out]
    n172 = shared-variable "NI-sbRIO9606-018BB5CF\\User-Defined Variables\\Axis 3.DIO Status (Port A)"(w313) -> ()  [unwired: 1 in, 1 out]
    n173 = shared-variable "NI-sbRIO9606-018BB5CF\\User-Defined Variables\\Axis 4.DIO Status (Port A)"(w312) -> ()  [unwired: 1 in, 1 out]
    n174 = shared-variable "NI-sbRIO9606-018BB5CF\\User-Defined Variables\\Axis 5.DIO Status (Port A)"(w311) -> ()  [unwired: 1 in, 1 out]
  }
  n175 = timed-loop "Reset Monitoring Loop" {
    timing: w4 -> [_]
    timing-out: [_] -> w3
    stop <- FALSE stop-if-true
    n176 = global read "Global FPGA.vi" "Reset Pending"() -> (w345:bool[])
    n177 = xnode "FPGA I/O Node"() -> ("Scan Clock"=w344:bool)  [unwired: 1 in, 1 out]
    n178 = feedback-in #1(w344) -> ()
    n179 = feedback #1() -> (w343:bool)  [unwired: 1 in]
    n180 = Greater?(x=w344, y=w343) -> (0:w349:bool)
    n181 = feedback #2() -> (w348:bool[])  [unwired: 1 in]
    n182 = Select(t=w345, s=w349, f=w348) -> (s? t:f=w346:bool[])
    n183 = feedback-in #2(w346) -> ()
    n184 = global write "Global FPGA.vi" "Reset"(w346) -> ()
  }
  n185 = node-c288(w3) -> ()
  n186 = node-c288(w5) -> ()
  n187 = node-c288(w7) -> ()
